vi "Statusword Decode.vi"(11 "Statusword U16":u16) -> (1 "Found":bool, 2 "Statusword out":T1, 3 "Statusword":T2, 5 "address":u16 format="%04x")   [LabVIEW 2016, in "IgusMotorDrive.lvclass"]
uses:
  IgusMotorDrive.lvclass
  typedefs/Statusword--enum.ctl
  typedefs/Statusword--cluster.ctl
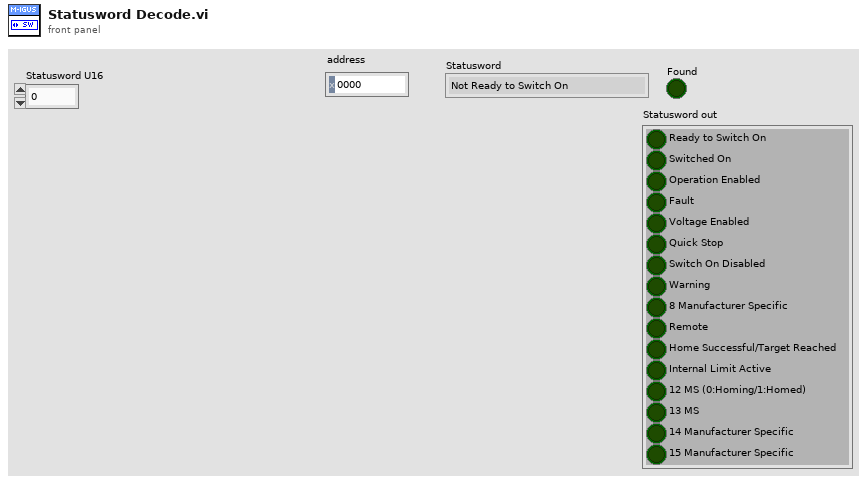
[diagram p1: front panel]
types:
  T1 = typedef "IgusMotorDrive.lvclass/Statusword--cluster.ctl" = cluster{"Ready to Switch On":bool, "Switched On":bool, "Operation Enabled":bool, "Fault":bool, "Voltage Enabled":bool, "Quick Stop":bool, "Switch On Disabled":bool, "Warning":bool, "8 Manufacturer Specific":bool, "Remote":bool, "Home Successful/Target Reached":bool, "Internal Limit Active":bool, "12 MS (0:Homing/1:Homed)":bool, "13 MS":bool, "14 Manufacturer Specific":bool, "15 Manufacturer Specific":bool}
  T2 = typedef "IgusMotorDrive.lvclass/Statusword--enum.ctl" = enum16{"Not Ready to Switch On", "Switch On Disabled", "Ready to Switch On", "Switched On", "Operation Enabled", "Quick Stop Active", "Fault Reaction Active", "Fault", "<Unknown>"}
  T3 = cluster{"Boolean array[0]":bool, "Boolean array[1]":bool, "Boolean array[2]":bool, "Boolean array[3]":bool, "Boolean array[4]":bool, "Boolean array[5]":bool, "Boolean array[6]":bool, "Boolean array[7]":bool, "Boolean array[8]":bool, "Boolean array[9]":bool, "Boolean array[10]":bool, "Boolean array[11]":bool, "Boolean array[12]":bool, "Boolean array[13]":bool, "Boolean array[14]":bool, "Boolean array[15]":bool}
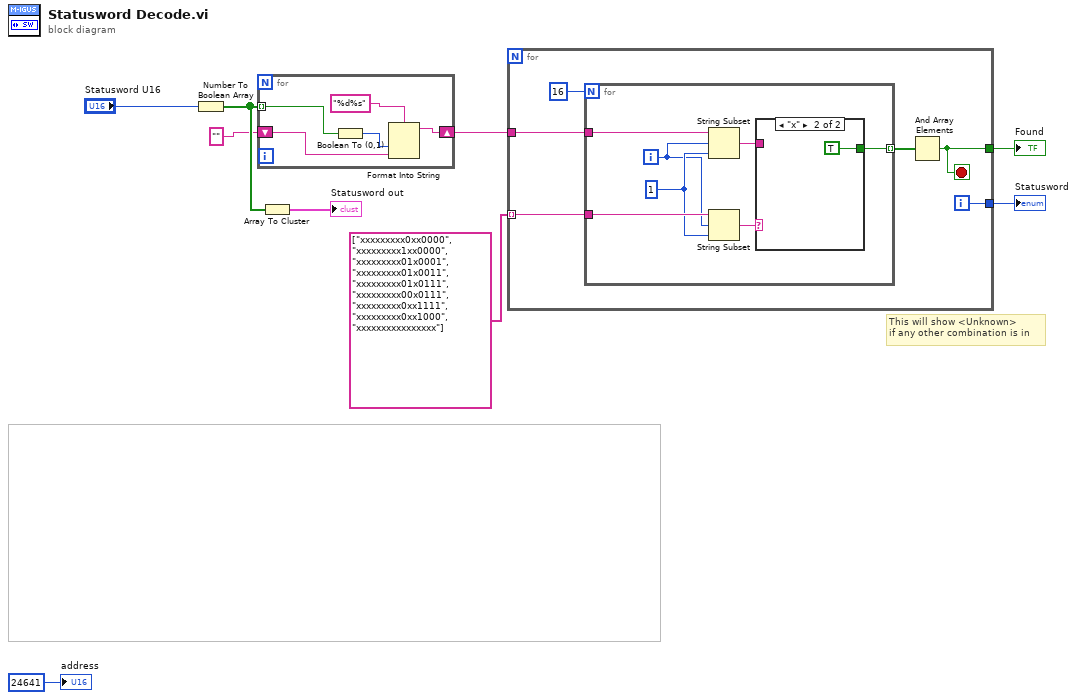
[diagram p0: block diagram]
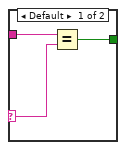
[diagram p2: hidden frame]
diagram:
  # "This will show <Unknown>\nif any other combination is in"
  n1 = Number To Boolean Array(number="Statusword U16") -> (Boolean array=w7:bool[])
  n2 = for {
    tunnel: w7 -> [w14] mode=indexing
    shift-right: [w10] -> w1
    shift-left: "" -> [w11]
    n3 = Boolean To (0,1)(Boolean=w14) -> (0, 1=w12:i16)
    n4 = Format Into String(format string="%d%s", w12, w11) -> (resulting string=w10:string)  [unwired: 2 in, 1 out]
  }
  n5 = Array To Cluster(array=w7) -> (cluster=→"Statusword out":T3)
  n6 = for {
    tunnel: w1 -> [w16]
    tunnel: string[] ["xxxxxxxxx0xx0000", "xxxxxxxxx1xx0000", "xxxxxxxxx01x0001", "xxxxxxxxx01x0011", "xxxxxxxxx01x0111", "xxxxxxxxx00x0111", "xxxxxxxxx0xx1111", "xxxxxxxxx0xx1000", "xxxxxxxxxxxxxxxx"] -> [w15] mode=indexing
    tunnel: [w20] -> w2
    tunnel: [w17] -> w4
    i -> [w20]
    stop <- w17 stop-if-true
    n7 = for {
      N: 16 -> [_]
      tunnel: w15 -> [w27]
      tunnel: w16 -> [w26]
      tunnel: [w23] -> w18 mode=indexing
      i -> [w24]
      w25 = 1 ("length (rest)")
      n8 = String Subset(string=w26, offset (0)=w24, length (rest)=w25) -> (substring=w21:string)
      n9 = String Subset(string=w27, offset (0)=w24, length (rest)=w25) -> (substring=w22:string)
      n10 = case shown="\"x\"" w22 {
        selector: w22 -> [w28 _]
        tunnel: [w30 TRUE] -> w23
        tunnel: w21 -> [w29 _]
        frame Default {
          n11 = Equal?(x=w29, y=w28) -> (x = y?=w30:bool)
        }
        frame "x" {
        }
      }
    }
    n12 = And Array Elements(Boolean array=w18) -> (logical AND=w17:bool)
  }
  "Statusword" <- w2
  "Found" <- w4
  "address" <- u16 24641 ("address")
